vi "transition_count.vi"(4 "previous_state":T1, 6 "current_state":T1, 8 "error in (no error)":errorcluster, 9 "step":string, 10 "index in":i32, 11 "recipe_data in":variant) -> (0 "error out":errorcluster, 2 "index out":i32, 3 "recipe_data out":variant)   [LabVIEW 2015, in "lv-recipe-machine.lvlib" / "example_01.lvlib"]
doc: "transition_count.vi will provide transition functionality for the count recipe."
uses:
  example_01.lvlib
  public/_controls/automatic_state.ctl
  lv-recipe-machine.lvlib
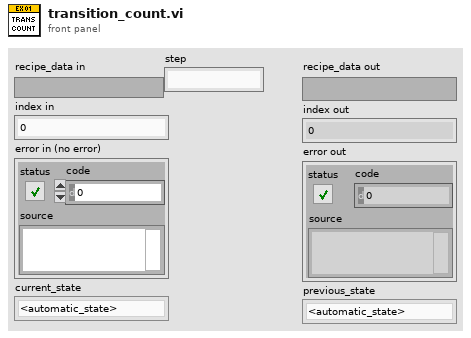
[diagram p1: front panel]
types:
  T1 = typedef "lv-recipe-machine.lvlib/automatic_state.ctl" = enum16{"<automatic_state>", "failed", "idle", "running", "paused", "stopped", "<null>"}
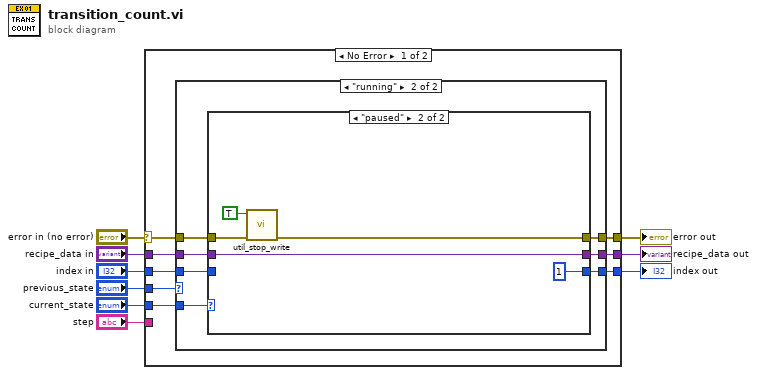
[diagram p0: block diagram]
diagram:
  n1 = case shown="No Error" "error in (no error)" {
    selector: "error in (no error)" -> [w15 w45]
    tunnel: [w14 w45] -> w8
    tunnel: "recipe_data in" -> [w13 w44]
    tunnel: "index in" -> [w11 w43]
    tunnel: "current_state" -> [w16 _]
    tunnel: "previous_state" -> [w17 _]
    tunnel: [w12 w44] -> w3
    tunnel: [w10 w43] -> w2
    tunnel: "step" -> [_ _]
    frame No Error {
      n2 = case shown="\"running\"" w17 {
        tunnel: w16 -> [w24 w34]
        tunnel: w15 -> [w21 w31]
        tunnel: [w20 w30] -> w14
        tunnel: w13 -> [w23 w33]
        tunnel: [w22 w32] -> w12
        tunnel: w11 -> [w19 w29]
        tunnel: [w18 w28] -> w10
        frame Default {
          n3 = case shown="Default" w24 {
            tunnel: w23 -> [w27]
            tunnel: [w27] -> w22
            tunnel: w21 -> [w26]
            tunnel: [w26] -> w20
            tunnel: w19 -> [w25]
            tunnel: [w25] -> w18
            frame Default {
            }
          }
        }
        frame "running" {
          n4 = case shown="\"paused\"" w34 {
            tunnel: w33 -> [w37 w42]
            tunnel: [w37 w42] -> w32
            tunnel: w31 -> [w36 w40]
            tunnel: [w36 w38] -> w30
            tunnel: w29 -> [w35 _]
            tunnel: [w35 1 ("index in")] -> w28
            frame Default {
            }
            frame "paused" {
              n5 = call "util_stop_write.vi"("error in (no error)"=w40, "stop"=TRUE) -> ("error out"=w38:errorcluster)  [unwired: 9 in]
            }
          }
        }
      }
    }
    frame Error {
    }
  }
  "error out" <- w8
  "recipe_data out" <- w3
  "index out" <- w2
